vi "UTILITY Modbus 1bit Number Combine.vi"(11 "register values":u16[](array[numeric])) -> (3 "Data":u16)   [LabVIEW 2016]
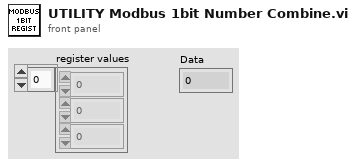
[diagram p1: front panel]
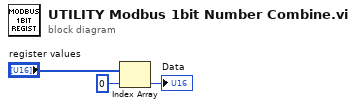
[diagram p0: block diagram]
diagram:
  n1 = Index Array(array="register values", index=0) -> (element=→"Data":u16)
